vi "XNET Example IP Stack Config - Single Interface.vi"(0 "XNET interface":refnum<k21>, 1 "is tagged?":bool, 2 "VLAN ID":u16, 5 "IPv4 address":string, 7 "IPv4 subnet mask":string, 9 "IPv6 address":string, 11 "error in (no error)":errorcluster) -> (4 "config":string, 15 "error out":errorcluster)   [LabVIEW 2018]
doc: "This example subVI generates a JSON configuration string for use with XNET IP Stack Create.vi. The configuration string supports a single XNET interface (physical interface), single VLAN (virtual interface), a single static IPv4 address, and a single static IPv6 address.\nYou can re-use this subVI in one of two ways: a) copy the subVI from the example diagram to your VI diagram, which re-uses the subVI unchanged (located in the XNET library), or b) Save As a copy of the subVI to your application folder, and change as needed."
uses:
  XNET Example IP Stack Config - Stack.ctl
  XNET Example IP Stack Config - XNET Interface.ctl
  XNET Example IP Stack Config - MAC.ctl
  XNET Example IP Stack Config - VLAN.ctl
  XNET Example IP Stack Config - Static Address.ctl
  XNET Example IP Stack Config - Static IPv6 Address.ctl
  XNET Example IP Stack Config - Proxy Server.ctl
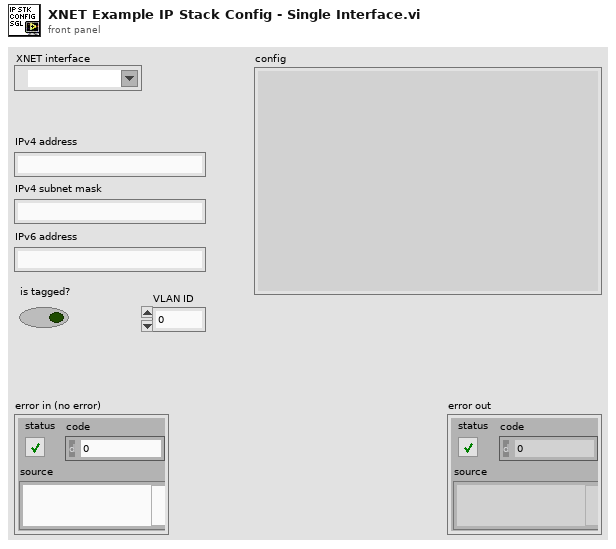
[diagram p1: front panel]
types:
  T1 = typedef "XNET Example IP Stack Config - VLAN.ctl" = cluster{"name":string, "isTagged":bool, "id":u16, "IPv4":cluster{"mode":string, "staticAddresses":T2[]}, "IPv6":cluster{"mode":string, "staticAddresses":T3[]}}
  T2 = typedef "XNET Example IP Stack Config - Static Address.ctl" = cluster{"address":string, "subnetMask":string}
  T3 = typedef "XNET Example IP Stack Config - Static IPv6 Address.ctl" = cluster{"address":string}
  T4 = typedef "XNET Example IP Stack Config - MAC.ctl" = cluster{"address":string, "VLANs":T1[]}
  T5 = typedef "XNET Example IP Stack Config - XNET Interface.ctl" = cluster{"name":string, "MACs":T4[]}
  T6 = typedef "XNET Example IP Stack Config - Stack.ctl" = cluster{"schema":string, "xnetInterfaces":T5[], "proxyServers":T7[]}
  T7 = typedef "XNET Example IP Stack Config - Proxy Server.ctl" = cluster{"protocol":string, "direction":string, "listenAddress":string, "listenPort":u16, "forwardingDestinationAddress":string, "forwardingDestinationPort":u16, "forwardingSourceAddress":string, "forwardingSourcePort":u16}
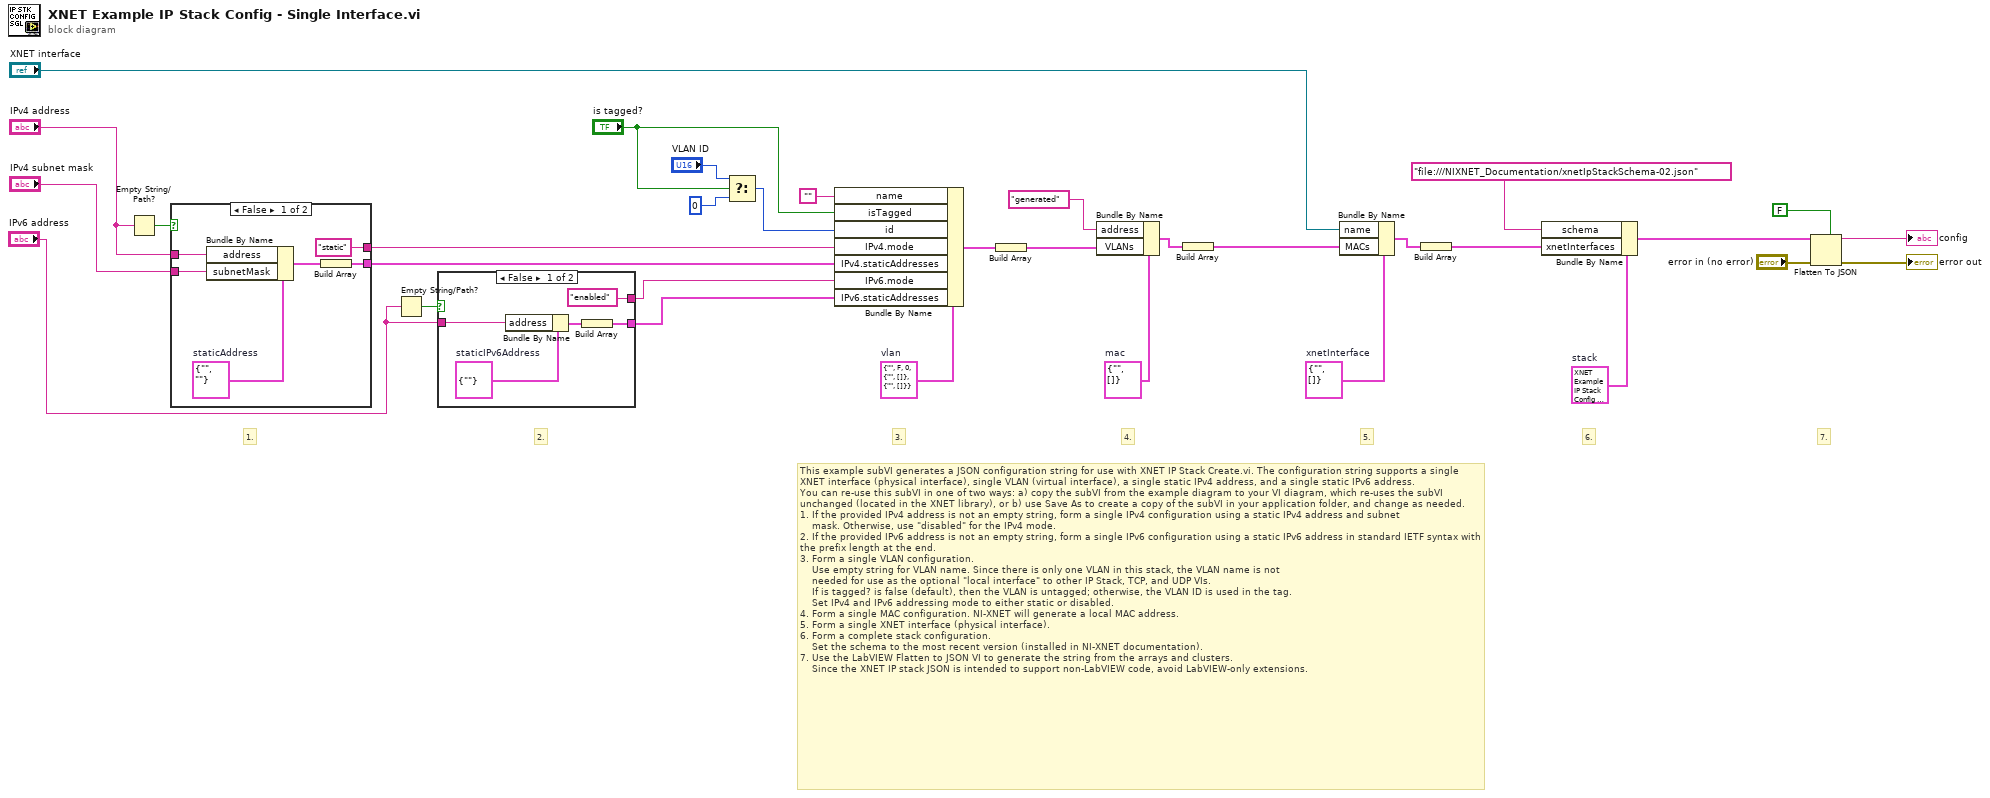
[diagram p0: block diagram]
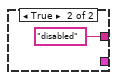
[diagram p2: hidden frame]
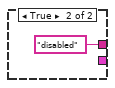
[diagram p3: hidden frame]
diagram:
  w16 = T1 {"name"="", "isTagged"=FALSE, "id"=0, "IPv4"={"mode"="", "staticAddresses"=[]}, "IPv6"={"mode"="", "staticAddresses"=[]}}  # vlan
  w21 = T4 {"address"="", "VLANs"=[]}  # mac
  w24 = T5 {"name"="", "MACs"=[]}  # xnetInterface
  w25 = T6 {"schema"="", "xnetInterfaces"=[{"name"="", "MACs"=[{"address"="", "VLANs"=[{"name"="", "isTagged"=FALSE, "id"=0, "IPv4"={"mode"="static", "staticAddresses"=[]}, "IPv6"={"mode"="", "staticAddresses"=[]}}]}]}], "proxyServers"=[]}  # stack
  # "2."
  # "7."
  # "6."
  # "5."
  # "4."
  # "3."
  # "This example subVI generates a JSON configuration string for use with XNET IP Stack Create.vi. The configuration string supports a single XNET interface (physical interface), single VLAN (virtual interface), a single static IPv4 address, and a single static IPv6 address.\nYou can re-use this subVI in one of two ways: a) copy the subVI from the example diagram to your VI diagram, which re-uses the subVI unchanged (located in the XNET library), or b) use Save As to create a copy of the subVI in your application folder, and change as needed.\n1. If the provided IPv4 address is not an empty string, form a single IPv4 configuration using a static IPv4 address and subnet\n    mask. Otherwise, use \"disabled\" for the IPv4 mode.\n2. If the provided IPv6 address is not an empty string, form a single IPv6 configuration using a static IPv6 address in standard IETF syntax with the prefix length at the end.\n3. Form a single VLAN configuration.\n    Use empty string for VLAN name. Since there is only one VLAN in this stack, the VLAN name is not\n    needed for use as the optional \"local interface\" to other IP Stack, TCP, and UDP VIs.\n    If is tagged? is false (default), then the VLAN is untagged; otherwise, the VLAN ID is used in the tag.\n    Set IPv4 and IPv6 addressing mode to either static or disabled.\n4. Form a single MAC configuration. NI-XNET will generate a local MAC address.\n5. Form a single XNET interface (physical interface).\n6. Form a complete stack configuration.\n    Set the schema to the most recent version (installed in NI-XNET documentation).\n7. Use the LabVIEW Flatten to JSON VI to generate the string from the arrays and clusters.\n    Since the XNET IP stack JSON is intended to support non-LabVIEW code, avoid LabVIEW-only extensions."
  # "1."
  n1 = Empty String/Path?(string/path="IPv4 address") -> (empty?=w6:bool)
  n2 = case shown="False" w6 {
    tunnel: [w36 _] -> w14
    tunnel: "IPv4 subnet mask" -> [w35 _]
    tunnel: "IPv4 address" -> [w34 _]
    tunnel: ["static" ("IPv4.mode") "disabled" ("IPv4.mode")] -> w7
    frame False {
      w37 = T2 {"address"="", "subnetMask"=""}  # staticAddress
      n3 = Bundle By Name(cluster=w37, "address"=w34, "subnetMask"=w35) -> (w38:T2)
      n4 = Build Array(w38) -> (w36:T2[])
    }
    frame True {
    }
  }
  n5 = Empty String/Path?(string/path="IPv6 address") -> (empty?=w4:bool)
  n6 = case shown="False" w4 {
    tunnel: "IPv6 address" -> [w40 _]
    tunnel: [w44 _] -> w2
    tunnel: ["enabled" ("IPv4.mode") "disabled" ("IPv4.mode")] -> w1
    frame False {
      w42 = T3 {"address"=""}  # staticIPv6Address
      n7 = Bundle By Name(cluster=w42, "address"=w40) -> (w41:T3)
      n8 = Build Array(w41) -> (w44:T3[])
    }
    frame True {
    }
  }
  n9 = Select(t="VLAN ID", s="is tagged?", f=u16 0) -> (s? t:f=w9:u16)
  n10 = Bundle By Name(cluster=w16, "name"="", "isTagged"="is tagged?", "id"=w9, "IPv4.mode"=w7, "IPv4.staticAddresses"=w14, "IPv6.mode"=w1, "IPv6.staticAddresses"=w2) -> (w18:T1)
  n11 = Build Array(w18) -> (w17:T1[])
  n12 = Bundle By Name(cluster=w21, "address"="generated" ("MAC address"), "VLANs"=w17) -> (w22:T4)
  n13 = Build Array(w22) -> (w20:T4[])
  n14 = Bundle By Name(cluster=w24, "name"="XNET interface", "MACs"=w20) -> (w23:T5)
  n15 = Build Array(w23) -> (w26:T5[])
  n16 = Bundle By Name(cluster=w25, "schema"="file:///NIXNET_Documentation/xnetIpStackSchema-02.json", "xnetInterfaces"=w26) -> (w28:T6)
  n17 = Flatten To JSON(enable LabVIEW extensions? (T)=FALSE, anything=w28, error in (no error)="error in (no error)") -> (JSON string=→"config":string, 11:→"error out":errorcluster)
